vi "SetAttributeViBoolean_ACP_CL_DD.vi"(7 "AttributeValue (Off)":bool, 8 "error in (no error)":errorcluster {"code" format="%.0x"}, 9 "AttributeID":u32(ring)=1150011 items=["ACP_AVERAGE_ENABLED"=1150011, "ACP_CARRIER_REFERENCE_FREQUENCY_AUTO_ENABLED"=1150016, "ACP_CARRIER_REFERENCE_LEVEL_AUTO_ENABLED"=1150018, "ACP_CARRIER_REFERENCE_NUMBER_AUTO_ENABLED"=1150020, "ACP_DETECTOR_AUTO_ENABLED"=1150058, "ACP_DISPLAY_BAR_GRAPH_ENABLED"=1150089, "ACP_DISPLAY_WINDOWY_AUTO_SCALE_ENABLED"=1150093, "ACP_FREQUENCY_PHASE_NOISE_OPTION_AUTO_ENABLED"=1150072, "ACP_LIMIT_TEST_ENABLED"=1150005, "ACP_MARKER_COUPLE_ENABLED"=1150098, "ACP_MARKER_ENABLED"=1150100, "ACP_NOISE_CORRECTION_ENABLED"=1150008, "ACP_OFFSET_FILTER_ENABLED"=1150104, "ACP_SWEEPCOUPLING_RESOLUTION_BANDWIDTH_AUTO_ENABLED"=1150024, "ACP_SWEEPCOUPLING_SWEEP_TIME_AUTO_ENABLED"=1150028, "ACP_SWEEPCOUPLING_VIDEO_BANDWIDTH_AUTO_ENABLED"=1150033, "ANALOG_ANTI_ALIASING_FILTER_AUTO_ENABLED"=1191707, "AUTO_SCALE_ENABLED"=1191693, "DIGITAL_DEMOD_AVERAGE_ENABLED"=1191758, "DIGITAL_DEMOD_CPM_AUTO_ENABLED"=1191643, "DIGITAL_DEMOD_DISPLAY_WINDOW_X_AUTO_SCALE_ENABLED"=1191608, "DIGITAL_DEMOD_EQUALIZATION_ENABLED"=1191633, "DIGITAL_DEMOD_EQUALIZATION_HOLD_ENABLED"=1191635, "DIGITAL_DEMOD_FSK_DEVIATION_REFERENCE_AUTO_ENABLED"=1191639, "DIGITAL_DEMOD_IF_GAIN"=1191656, "DIGITAL_DEMOD_IF_GAIN_AUTO_ENABLED"=1191657, "DIGITAL_DEMOD_IQ_NORMALIZATION_ENABLED"=1191645, "DIGITAL_DEMOD_IQ_OFFSET_COMPENSATION_ENABLED"=1191663, "DIGITAL_DEMOD_LIMIT_TEST_ENABLED"=1191612, "DIGITAL_DEMOD_LOW_SNR_ENHANCEMENT_ENABLED"=1191649, "DIGITAL_DEMOD_MARKER_COUPLE_ENABLED"=1191606, "DIGITAL_DEMOD_MARKER_ENABLED"=1191597, "DIGITAL_DEMOD_MULTI_CARRIER_FILTER_ENABLED"=1191679, "DIGITAL_DEMOD_QUAD_SKEW_COUPLING_ENABLED"=1191644, "DIGITAL_DEMOD_SYNC_BURST_SEARCH_ENABLED"=1191654, "DIGITAL_DEMOD_SYNC_SEARCH_ENABLED"=1191651, "DIGITAL_DEMOD_TRACE_LIMIT_DISPLAY_ENABLED"=1191669, "DIGITAL_DEMOD_TRACE_LIMIT_MARGIN_AUTO_ENABLED"=1191675, "FREQUENCY_CENTER_STEP_AUTO_ENABLED"=1150134, "GATING_ENABLED"=1190015, "GATING_HOLD_OFF_TIME_AUTO_ENABLED"=1150143, "GATING_VIEW"=1190020, "INPUT_IQ_I_DIFFERENTIAL_ENABLED"=1191713, "INPUT_IQ_MIRROR_ENABLED"=1191712, "INPUT_IQ_Q_DIFFERENTIAL_ENABLED"=1191714, "INPUT_RF_PRE_AMP_ENABLED"=1190117, "LEVEL_ELECTRONIC_ATTENUATION_STATE_ENABLED"=1190122, "SIMULATE"=1050005], 10 "RepCapIdentifier":string, 11 "instrument handle":refnum<k15>) -> (0 "error out":errorcluster {"code" format="%.0x"}, 3 "instrument handle out":refnum<k15>)   [LabVIEW 2021, in "Keysight XSAnVMA.lvlib"]
doc: "Sets Boolean Attribute from instrumrnt driver.\nThe following attributes are supported:\n\nACP_AVERAGE_ENABLED\nACP_CARRIER_REFERENCE_FREQUENCY_AUTO_ENABLED\nACP_CARRIER_REFERENCE_LEVEL_AUTO_ENABLED\nACP_CARRIER_REFERENCE_NUMBER_AUTO_ENABLED\nACP_DETECTOR_AUTO_ENABLED\nACP_DISPLAY_BAR_GRAPH_ENABLED\nACP_DISPLAY_WINDOWY_AUTO_SCALE_ENABLED\nACP_FREQUENCY_PHASE_NOISE_OPTION_AUTO_ENABLED\nACP_LIMIT_TEST_ENABLED\nACP_MARKER_COUPLE_ENABLED\nACP_MARKER_ENABLED\nACP_NOISE_CORRECTION_ENABLED\nACP_OFFSET_FILTER_ENABLED\nACP_SWEEPCOUPLING_RESOLUTION_BANDWIDTH_AUTO_ENABLED\nACP_SWEEPCOUPLING_SWEEP_TIME_AUTO_ENABLED\nACP_SWEEPCOUPLING_VIDEO_BANDWIDTH_AUTO_ENABLED\nANALOG_ANTI_ALIASING_FILTER_AUTO_ENABLED\nAUTO_SCALE_ENABLED\nDIGITAL_DEMOD_AVERAGE_ENABLED\nDIGITAL_DEMOD_CPM_AUTO_ENABLED\nDIGITAL_DEMOD_DISPLAY_WINDOW_X_AUTO_SCALE_ENABLED\nDIGITAL_DEMOD_EQUALIZATION_ENABLED\nDIGITAL_DEMOD_EQUALIZATION_HOLD_ENABLED\nDIGITAL_DEMOD_FSK_DEVIATION_REFERENCE_AUTO_ENABLED\nDIGITAL_DEMOD_IF_GAIN\nDIGITAL_DEMOD_IF_GAIN_AUTO_ENABLED\nDIGITAL_DEMOD_IQ_NORMALIZATION_ENABLED\nDIGITAL_DEMOD_IQ_OFFSET_COMPENSATION_ENABLED\nDIGITAL_DEMOD_LIMIT_TEST_ENABLED\nDIGITAL_DEMOD_LOW_SNR_ENHANCEMENT_ENABLED\nDIGITAL_DEMOD_MARKER_COUPLE_ENABLED\nDIGITAL_DEMOD_MARKER_ENABLED\nDIGITAL_DEMOD_MULTI_CARRIER_FILTER_ENABLED\nDIGITAL_DEMOD_QUAD_SKEW_COUPLING_ENABLED\nDIGITAL_DEMOD_SYNC_BURST_SEARCH_ENABLED\nDIGITAL_DEMOD_SYNC_SEARCH_ENABLED\nDIGITAL_DEMOD_TRACE_LIMIT_DISPLAY_ENABLED\nDIGITAL_DEMOD_TRACE_LIMIT_MARGIN_AUTO_ENABLED\nFREQUENCY_CENTER_STEP_AUTO_ENABLED\nGATING_ENABLED\nGATING_HOLD_OFF_TIME_AUTO_ENABLED\nGATING_VIEW\nINPUT_IQ_I_DIFFERENTIAL_ENABLED\nINPUT_IQ_MIRROR_ENABLED\nINPUT_IQ_Q_DIFFERENTIAL_ENABLED\nINPUT_RF_PRE_AMP_ENABLED\nLEVEL_ELECTRONIC_ATTENUATION_STATE_ENABLED\nSIMULATE"
uses:
  <instrlib>/Keysight XSAnVMA/Keysight XSAnVMA.lvlib
  KtXSAnVMA_64.dll
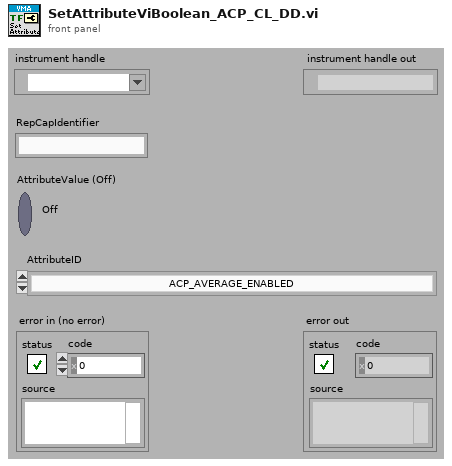
[diagram p1: front panel]
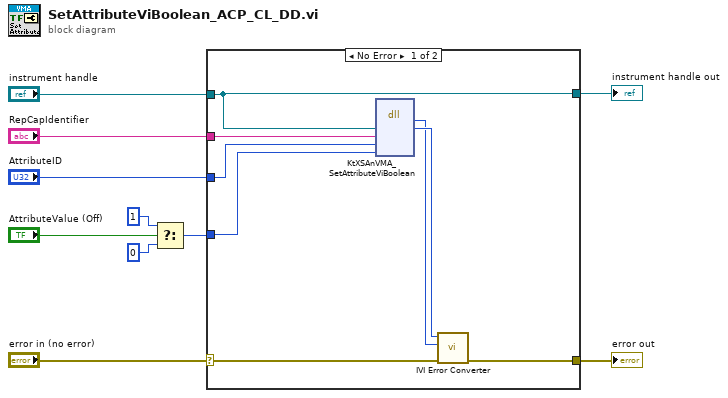
[diagram p0: block diagram]
diagram:
  n1 = Select(t=u16 1, s="AttributeValue (Off)", f=u16 0) -> (s? t:f=w3:u16)
  n2 = case shown="No Error" "error in (no error)" {
    selector: "error in (no error)" -> [w16 w20]
    tunnel: [w15 w20] -> w10
    tunnel: "instrument handle" -> [w11 w19]
    tunnel: "RepCapIdentifier" -> [w14 _]
    tunnel: "AttributeID" -> [w13 _]
    tunnel: w3 -> [w12 _]
    tunnel: [w11 w19] -> w1
    frame No Error {
      n3 = dll-call lib="KtXSAnVMA**.dll" fn="KtXSAnVMA_SetAttributeViBoolean"("Vi"=w11, "RepCapIdentifier"=w14, "AttributeID"=w13, "AttributeValue"=w12) -> ("return type"=w17:i32, "Vi"=w18:u32)  [unwired: 6 in, 2 out]
      n4 = call <instrlib>:"IVI Error Converter.vi"("error in (no error)"=w16, "IVI error code (0)"=w17, "instrument handle"=w18) -> ("error out"=w15:errorcluster)  [unwired: 7 in, 1 out]
    }
    frame Error {
    }
  }
  "error out" <- w10
  "instrument handle out" <- w1
